vi "VisitLVType.vi"(8 "error in (no error)":errorcluster, 10 "LVType":refnum<class "LVType.lvclass">, 11 "LVTypeVisitor in":refnum<class "LVTypeVisitor.lvclass">) -> (0 "error out":errorcluster, 3 "LVTypeVisitor out":refnum<class "LVTypeVisitor.lvclass">)   [LabVIEW 2020, in "LVDataTypes.lvlib" / "LVTypeVisitor.lvclass"]
uses:
  <vilib>/AppBuilder/Engine/WebServiceDescription/LVDataTypes/LVTypeVisitor/LVTypeVisitor.lvclass
  <vilib>/AppBuilder/Engine/WebServiceDescription/LVDataTypes/LVType/LVType.lvclass
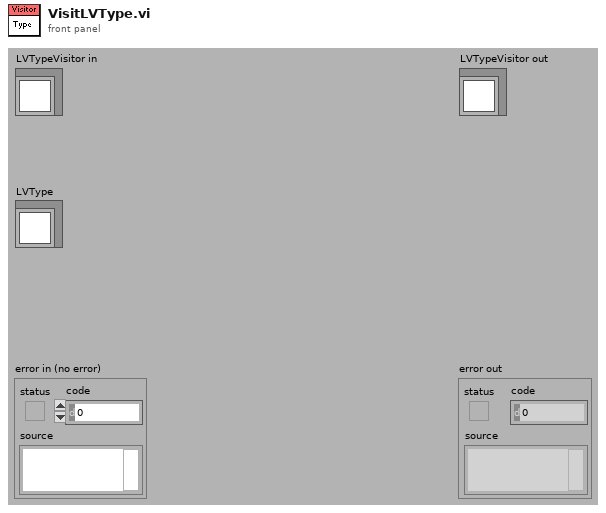
[diagram p1: front panel]
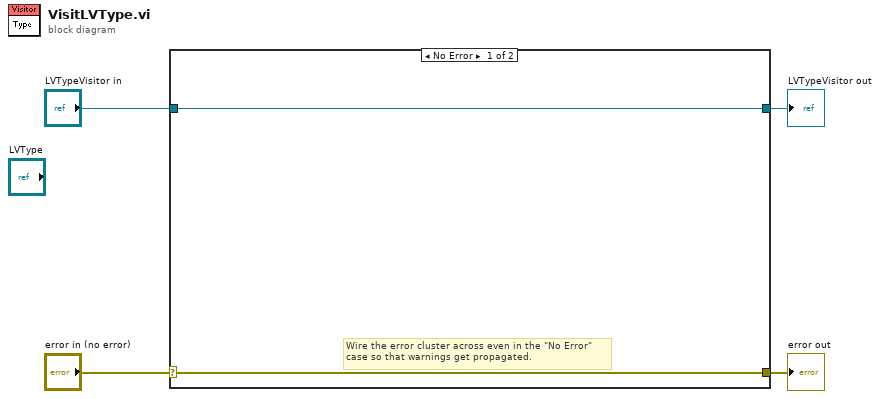
[diagram p0: block diagram]
diagram:
  n1 = case shown="No Error" "error in (no error)" {
    selector: "error in (no error)" -> [w5 w8]
    tunnel: [w5 w8] -> w3
    tunnel: [w6 w7] -> w1
    tunnel: "LVTypeVisitor in" -> [w6 w7]
    frame No Error {
      # "Wire the error cluster across even in the \"No Error\"\ncase so that warnings get propagated."
    }
    frame Error {
    }
  }
  "error out" <- w3
  "LVTypeVisitor out" <- w1
